vi "dynamic_calc_dual.vi"(0 "x  dist":dbl[](array[numeric])=[77911.0, 79996.0, 60540.0, 54460.0, 36220.0], 5 "Array 2":T2(array[cluster]), 11 "y  dist":dbl[](array[numeric])=[77911.0, 79996.0, 60540.0, 54460.0, 36220.0], 12 "DYNAMIC":T1(array[cluster]), 13 "DYNAMIC 2":T1(array[cluster])) -> (4 "dist":dbl[][](array[numeric]), 6 "time":dbl[][](array[numeric]))   [LabVIEW 2015]
panel:
  out "appended array":dbl[][](array[numeric])
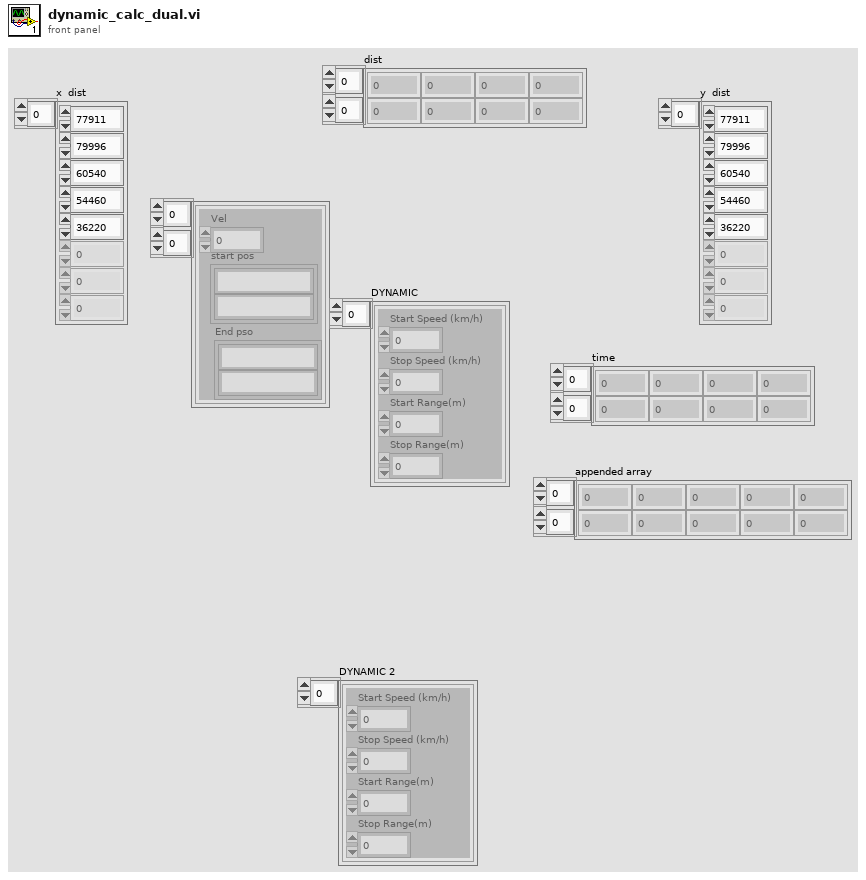
[diagram p1: front panel]
types:
  T1 = cluster{"Start Speed (km/h)":dbl, "Stop Speed (km/h) ":dbl, "Start Range(m)":dbl, "Stop Range(m)":dbl}[]
  T2 = cluster{"Vel":dbl, "start pos":cluster{string, string}, "End pso":cluster{string, string}}[][]
  T3 = cluster{"Vel":dbl, "start pos":cluster{string, string}, "End pso":cluster{string, string}}[]
  T4 = cluster{"Start Speed (km/h)":dbl, "Stop Speed (km/h) ":dbl, "Start Range(m)":dbl, "Stop Range(m)":dbl}
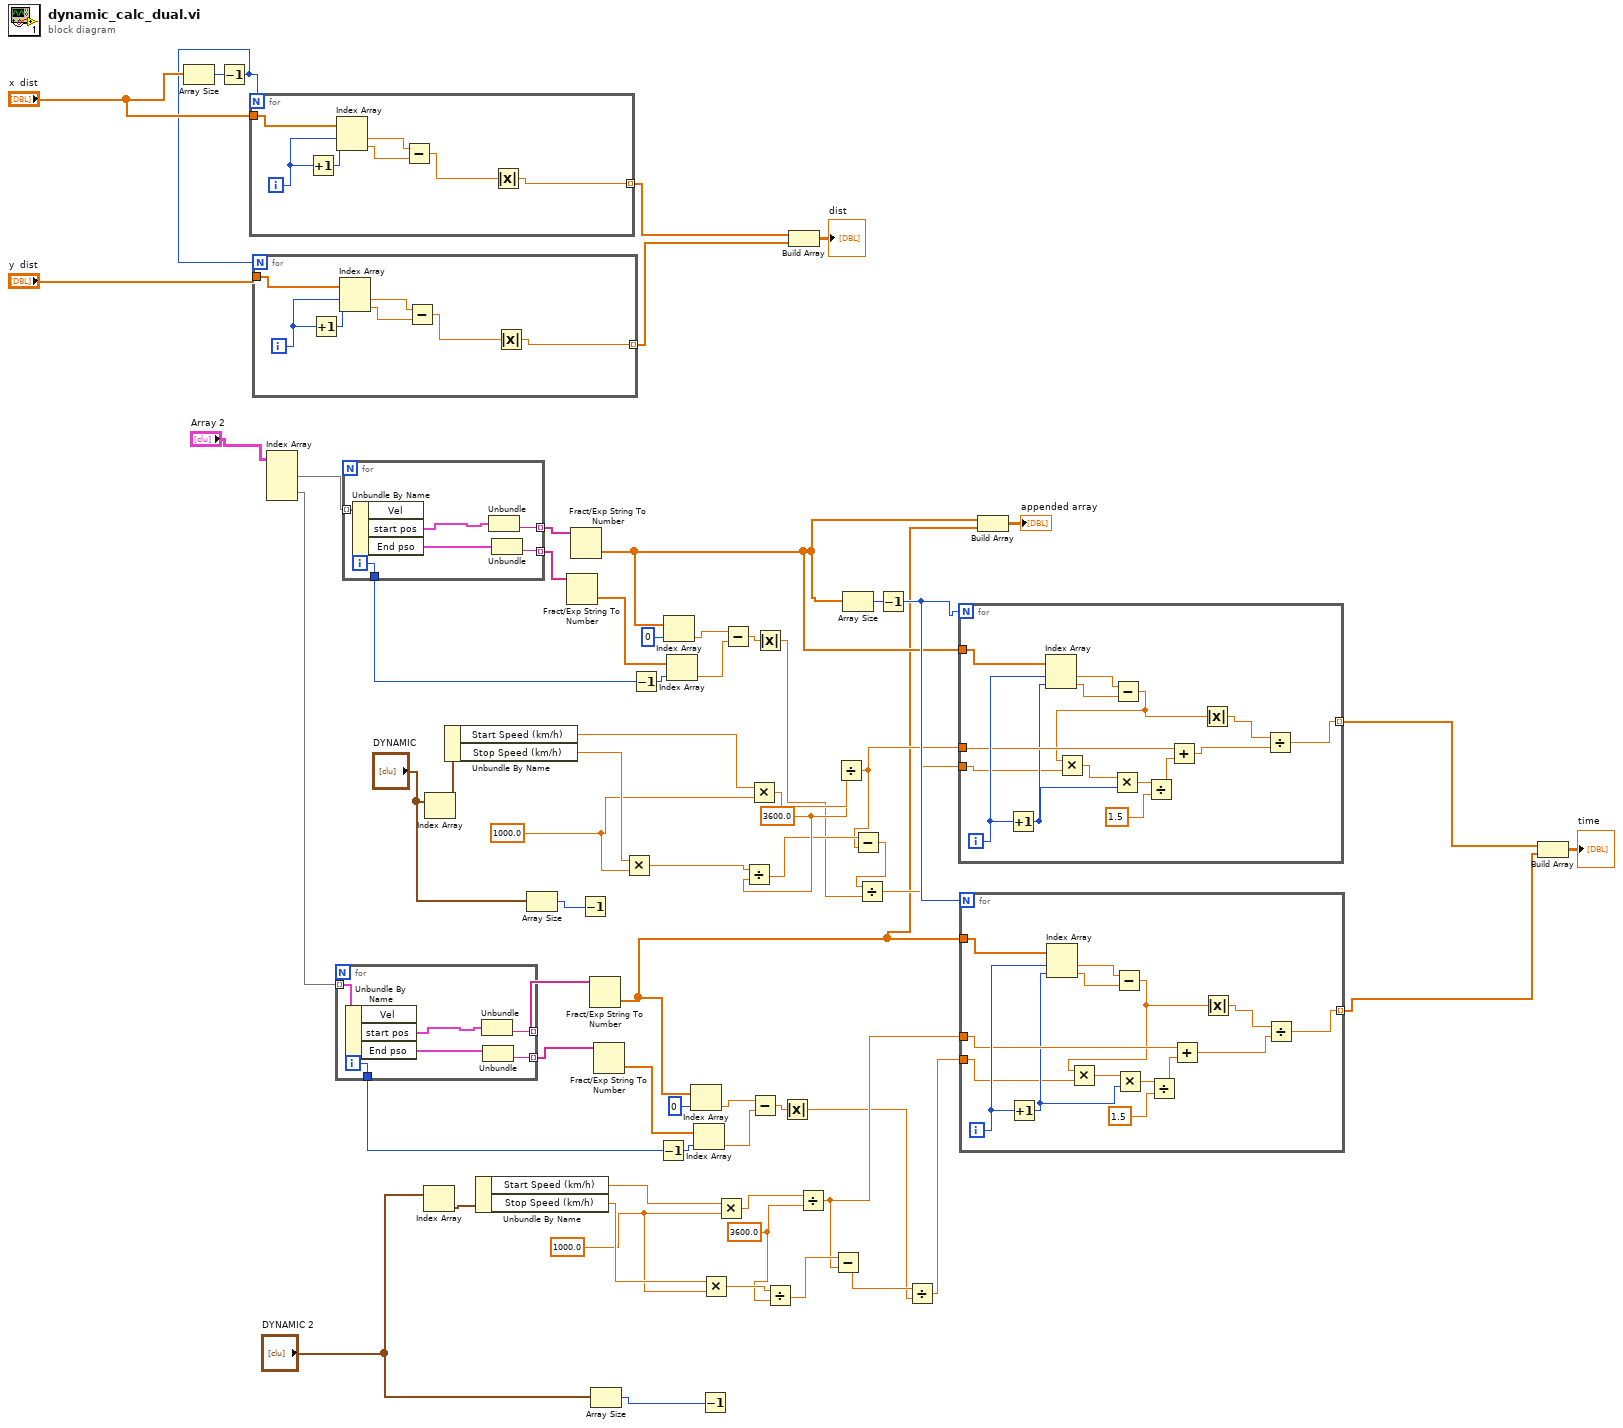
[diagram p0: block diagram]
diagram:
  w37 = 3600.0 ("y")
  w38 = 1000.0 ("y")
  w31 = 3600.0 ("y")
  w32 = 1000.0 ("y")
  n1 = Array Size(array="x  dist") -> (size(s)=w64:i32)
  n2 = Decrement(x=w64) -> (x-1=w47:i32)
  n3 = for {
    N: w47 -> [_]
    tunnel: "x  dist" -> [w71]
    tunnel: [w65] -> w46 mode=indexing
    i -> [w69]
    n4 = Increment(x=w69) -> (x+1=w70:i32)
    n5 = Index Array(array=w71, index #1=w69, index #2=w70) -> (element #1=w68:dbl, element #2=w67:dbl)
    n6 = Subtract(x=w68, y=w67) -> (x-y=w66:dbl)
    n7 = Absolute Value(x=w66) -> (abs(x)=w65:dbl)
  }
  n8 = for {
    N: w47 -> [_]
    tunnel: "y  dist" -> [w78]
    tunnel: [w72] -> w45 mode=indexing
    i -> [w76]
    n9 = Increment(x=w76) -> (x+1=w77:i32)
    n10 = Index Array(array=w78, index #1=w76, index #2=w77) -> (element #1=w75:dbl, element #2=w74:dbl)
    n11 = Subtract(x=w75, y=w74) -> (x-y=w73:dbl)
    n12 = Absolute Value(x=w73) -> (abs(x)=w72:dbl)
  }
  n13 = Index Array(array="Array 2") -> (element #1=w61:T3, element #2=w55:T3)  [unwired: 4 in]
  n14 = for {
    tunnel: [w83] -> w54 mode=indexing
    tunnel: w55 -> [w82] mode=indexing
    tunnel: [w80] -> w5 mode=indexing
    tunnel: [w79] -> w4
    i -> [w79]
    n15 = Unbundle By Name(w82) -> ("start pos"=w84:cluster{string, string}, "End pso"=w81:cluster{string, string})  [unwired: 1 out]
    n16 = Unbundle(w84) -> (w83:string)  [unwired: 1 out]
    n17 = Unbundle(w81) -> (w80:string)  [unwired: 1 out]
  }
  n18 = for {
    tunnel: w61 -> [w90] mode=indexing
    tunnel: [w88] -> w60 mode=indexing
    tunnel: [w86] -> w20 mode=indexing
    tunnel: [w85] -> w13
    i -> [w85]
    n19 = Unbundle By Name(w90) -> ("start pos"=w89:cluster{string, string}, "End pso"=w87:cluster{string, string})  [unwired: 1 out]
    n20 = Unbundle(w89) -> (w88:string)  [unwired: 1 out]
    n21 = Unbundle(w87) -> (w86:string)  [unwired: 1 out]
  }
  n22 = Index Array(array="DYNAMIC 2") -> (element=w43:T4)  [unwired: 1 in]
  n23 = Index Array(array="DYNAMIC") -> (element=w56:T4)  [unwired: 1 in]
  n24 = Unbundle By Name(w56) -> ("Start Speed (km/h)"=w58:dbl, "Stop Speed (km/h)"=w33:dbl)
  n25 = Unbundle By Name(w43) -> ("Start Speed (km/h)"=w42:dbl, "Stop Speed (km/h)"=w39:dbl)
  n26 = Array Size(array="DYNAMIC") -> (size(s)=w24:i32)
  n27 = Fract/Exp String To Number(string=w20) -> (number=w14:dbl[])  [unwired: 3 in, 1 out]
  n28 = Fract/Exp String To Number(string=w60) -> (number=w15:dbl[])  [unwired: 3 in, 1 out]
  n29 = Decrement(x=w24) -> ()  [unwired: 1 out]
  n30 = Fract/Exp String To Number(string=w54) -> (number=w3:dbl[])  [unwired: 3 in, 1 out]
  n31 = Array Size(array="DYNAMIC 2") -> (size(s)=w28:i32)
  n32 = Fract/Exp String To Number(string=w5) -> (number=w10:dbl[])  [unwired: 3 in, 1 out]
  n33 = Multiply(x=w33, y=w32) -> (x*y=w34:dbl)
  n34 = Decrement(x=w13) -> (x-1=w12:i32)
  n35 = Decrement(x=w4) -> (x-1=w11:i32)
  n36 = Index Array(array=w15, index=0) -> (element=w17:dbl)
  n37 = Index Array(array=w14, index=w12) -> (element=w18:dbl)
  n38 = Index Array(array=w3, index=0) -> (element=w8:dbl)
  n39 = Index Array(array=w10, index=w11) -> (element=w7:dbl)
  n40 = Decrement(x=w28) -> ()  [unwired: 1 out]
  n41 = Multiply(x=w39, y=w38) -> (x*y=w40:dbl)
  n42 = Multiply(x=w42, y=w38) -> (x*y=w41:dbl)
  n43 = Subtract(x=w17, y=w18) -> (x-y=w16:dbl)
  n44 = Divide(x=w34, y=w31) -> (x/y=w30:dbl)
  n45 = Multiply(x=w58, y=w32) -> (x*y=w57:dbl)
  n46 = Subtract(x=w8, y=w7) -> (x-y=w9:dbl)
  n47 = Absolute Value(x=w16) -> (abs(x)=w2:dbl)
  n48 = Divide(x=w40, y=w37) -> (x/y=w36:dbl)
  n49 = Absolute Value(x=w9) -> (abs(x)=w1:dbl)
  n50 = Build Array(w46, w45) -> (→"dist":dbl[][])
  n51 = Divide(x=w41, y=w37) -> (x/y=w35:dbl)
  n52 = Subtract(x=w36, y=w35) -> (x-y=w26:dbl)
  n53 = Divide(x=w57, y=w31) -> (x/y=w29:dbl)
  n54 = Array Size(array=w15) -> (size(s)=w59:i32)
  n55 = Subtract(x=w30, y=w29) -> (x-y=w22:dbl)
  n56 = Divide(x=w22, y=w2) -> (x/y=w21:dbl)
  n57 = Decrement(x=w59) -> (x-1=w53:i32)
  n58 = Divide(x=w26, y=w1) -> (x/y=w25:dbl)
  n59 = for {
    N: w53 -> [_]
    tunnel: w15 -> [w105]
    tunnel: [w100] -> w51 mode=indexing
    tunnel: w29 -> [w96]
    tunnel: w21 -> [w92]
    i -> [w104]
    n60 = Increment(x=w104) -> (x+1=w95:i32)
    n61 = Index Array(array=w105, index #1=w104, index #2=w95) -> (element #1=w103:dbl, element #2=w102:dbl)
    n62 = Subtract(x=w103, y=w102) -> (x-y=w93:dbl)
    n63 = Multiply(x=w93, y=w92) -> (x*y=w91:dbl)
    n64 = Multiply(x=w91, y=w95) -> (x*y=w99:dbl)
    n65 = Divide(x=w99, y=1.5) -> (x/y=w97:dbl)
    n66 = Add(x=w96, y=w97) -> (x+y=w94:dbl)
    n67 = Absolute Value(x=w93) -> (abs(x)=w101:dbl)
    n68 = Divide(x=w101, y=w94) -> (x/y=w100:dbl)
  }
  n69 = for {
    N: w53 -> [_]
    tunnel: w3 -> [w120]
    tunnel: [w115] -> w50 mode=indexing
    tunnel: w35 -> [w111]
    tunnel: w25 -> [w108]
    i -> [w119]
    n70 = Increment(x=w119) -> (x+1=w109:i32)
    n71 = Index Array(array=w120, index #1=w119, index #2=w109) -> (element #1=w118:dbl, element #2=w117:dbl)
    n72 = Subtract(x=w118, y=w117) -> (x-y=w107:dbl)
    n73 = Multiply(x=w107, y=w108) -> (x*y=w106:dbl)
    n74 = Multiply(x=w106, y=w109) -> (x*y=w114:dbl)
    n75 = Divide(x=w114, y=1.5) -> (x/y=w112:dbl)
    n76 = Add(x=w111, y=w112) -> (x+y=w110:dbl)
    n77 = Absolute Value(x=w107) -> (abs(x)=w116:dbl)
    n78 = Divide(x=w116, y=w110) -> (x/y=w115:dbl)
  }
  n79 = Build Array(w15, w3) -> (→"appended array":dbl[][])
  n80 = Build Array(w51, w50) -> (→"time":dbl[][])
